vi "sweeper.vi"() -> ()   [LabVIEW 2012]
uses:
  scan_info.ctl
  stimulus.ctl
  injection_point.ctl
  initialization/micron_globals.vi
  <vilib>/Analysis/1siggen.llb/Ramp Pattern by Samples.vi
  <vilib>/Analysis/NI_AALBase.lvlib
panel:
  in  "Axis mode":enum16{"Absolute axis", "Relative axis", "Pose"}(ring)
  in  "Motion axis":string(combo)
  out "Current point":dbl format="%#_3p"
  in  "1/x scaling":bool
  in  "stop":bool
  out "Sweeping":bool
  in  "Linear type":u16(ring) items=["Linear", "Logarithmic"]
  in  "Sweep info":T1 {"End" format="%#_3p"; "Start" format="%#_3p"}
  in  "Start sweep":bool
  in  "Manual":bool
  in  "Stimulus":T2={"Type"=enum."Off", "Phase"=0.0, "Amplitude"=[0.0, 0.0, 0.0, 0.0, 0.0, 0.0], "Injection point"=enum."Total pose", "Closed loop"=TRUE, "Offset"=[0.0, 0.0, 0.0, 0.0, 0.0, 0.0], "Tip -> world"=TRUE, "Frequency"=0.0, "Length"=0.0} {"Length" min=0.0 max=100.0 step=100.0 format="%#_4p"; "Frequency" min=0.0 step=100.0 format="%#_4g"; "Offset" format="%#_3p"; "Amplitude" format="%#_3p"; "Phase" min=-180.0 max=360.0 step=100.0 format="%#.2f"}
  in  "Scrollbar":sgl(c297)
  # "Sweeper"
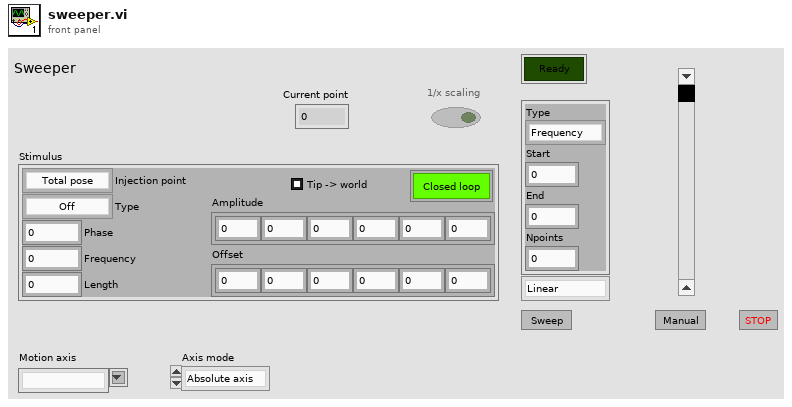
[diagram p1: front panel]
types:
  T1 = typedef "scan_info.ctl" = cluster{"Type":enum16{"Frequency", "Offset", "Motion"}, "Start":sgl, "End":sgl, "Npoints":i32}
  T2 = typedef "stimulus.ctl" = cluster{"Type":enum16{"Off", "Step", "Sine", "Triangle", "Arbitrary"}, "Phase":dbl, "Amplitude":sgl[], "Injection point":T3, "Closed loop":bool, "Offset":sgl[], "Tip -> world":bool, "Frequency":dbl, "Length":dbl}
  T3 = typedef "injection_point.ctl" = enum16{"Total pose", "V limiter", "Goal ", "Link position", "KF link position", "Inverse kin", "Link goal", "Link error", "Controller", "Output", "Drive", "Light"}
  T4 = enum8{"Enabled", "Disabled", "Disabled and Grayed Out"}
  T5 = typedef "ui_override_opts.ctl" = cluster{"Triggering":bool, "Parameters":bool, "Stimulus":bool, "Calibration":bool, "Modes":bool}
  T6 = typedef "Micron params.ctl" = cluster{"Stimulus":T2, "Goal Filter A":T7, "Mode controls":T8, "Manipulator type":enum16{"Current piezo", "Voltage piezo"}, "Manipulator calibration":T9, "Network":T11, "Goal Filter B":T7, "Cancellation":T12, "Transition time":sgl, "Estimation":T14}
  T7 = typedef "goal_loop_parms.ctl" = cluster{"Speedup max":sgl, "Speedup thresh":sgl, "Speedup nonlin":sgl, "Filters":cluster{"Lower Fc":sgl, "Lower Q":sgl, "Scale factor":sgl, "Upper Fc":sgl, "Upper Q":sgl, "V limit":sgl, "V limit range":sgl}[]}
  T8 = typedef "mode_conrols.ctl" = cluster{"Hold":bool, "Cancellation":bool, "Goal filter":bool, "Trigger":bool}
  T9 = typedef "manipulator_cal.ctl" = cluster{"Tool offsets":sgl[][], "Tip light calibration":T10, "Handle light calibration":T10, "Base pivots":sgl[][], "Output pivots":sgl[][], "Length center":sgl, "Workspace height":sgl[], "Workspace diameter":sgl[], "Linearization":sgl[][], "Stack travel":sgl, "Saturation pos":sgl, "Inverse filters":cluster{"filter structure":enum32{"IIR 2nd Order", "IIR 4th Order"}, "Reverse Coefficients":dbl[], "Forward Coefficients":dbl[]}[]}
  T10 = typedef "probe_calibration.ctl" = sgl[][]
  T11 = typedef "network_params.ctl" = cluster{"Remote Host":string, "Send Status":bool, "Send Port":u16, "Recv Commands":bool, "Recv Port":u16}
  T12 = typedef "sq_control_params.ctl" = cluster{"KP":T13, "KI":sgl, "KD":T13, "Max vel":sgl, "Max acc":sgl, "Int error limit":sgl, "RCM gain":sgl, "Bypass":bool, "Degraded gain":sgl}
  T13 = typedef "decoupled_gain.ctl" = cluster{"XY":sgl, "Rxy":sgl, "Z":sgl, "Rz":sgl}
  T14 = typedef "estimation_controls.ctl" = cluster{"Link":cluster{"Measure noise":dbl[], "Process noise":dbl[], "Alt process noise":dbl[], "Alt turnoff cycles":i32, "Innovation limit":dbl[], "Residue threshold":dbl, "Enable":bool}, "Handle":cluster{"Measure noise":dbl[], "Process noise":dbl[], "State limits":dbl[], "Innovation limit":dbl[], "Prediction Lookahead":sgl, "Enable":bool}}
  T15 = typedef "motion_status.ctl" = cluster{"Axis names":string[], "Axis positions":dbl[], "Pose":dbl[], "Timestamp":u32, "Ready":bool, "Stopped":bool}
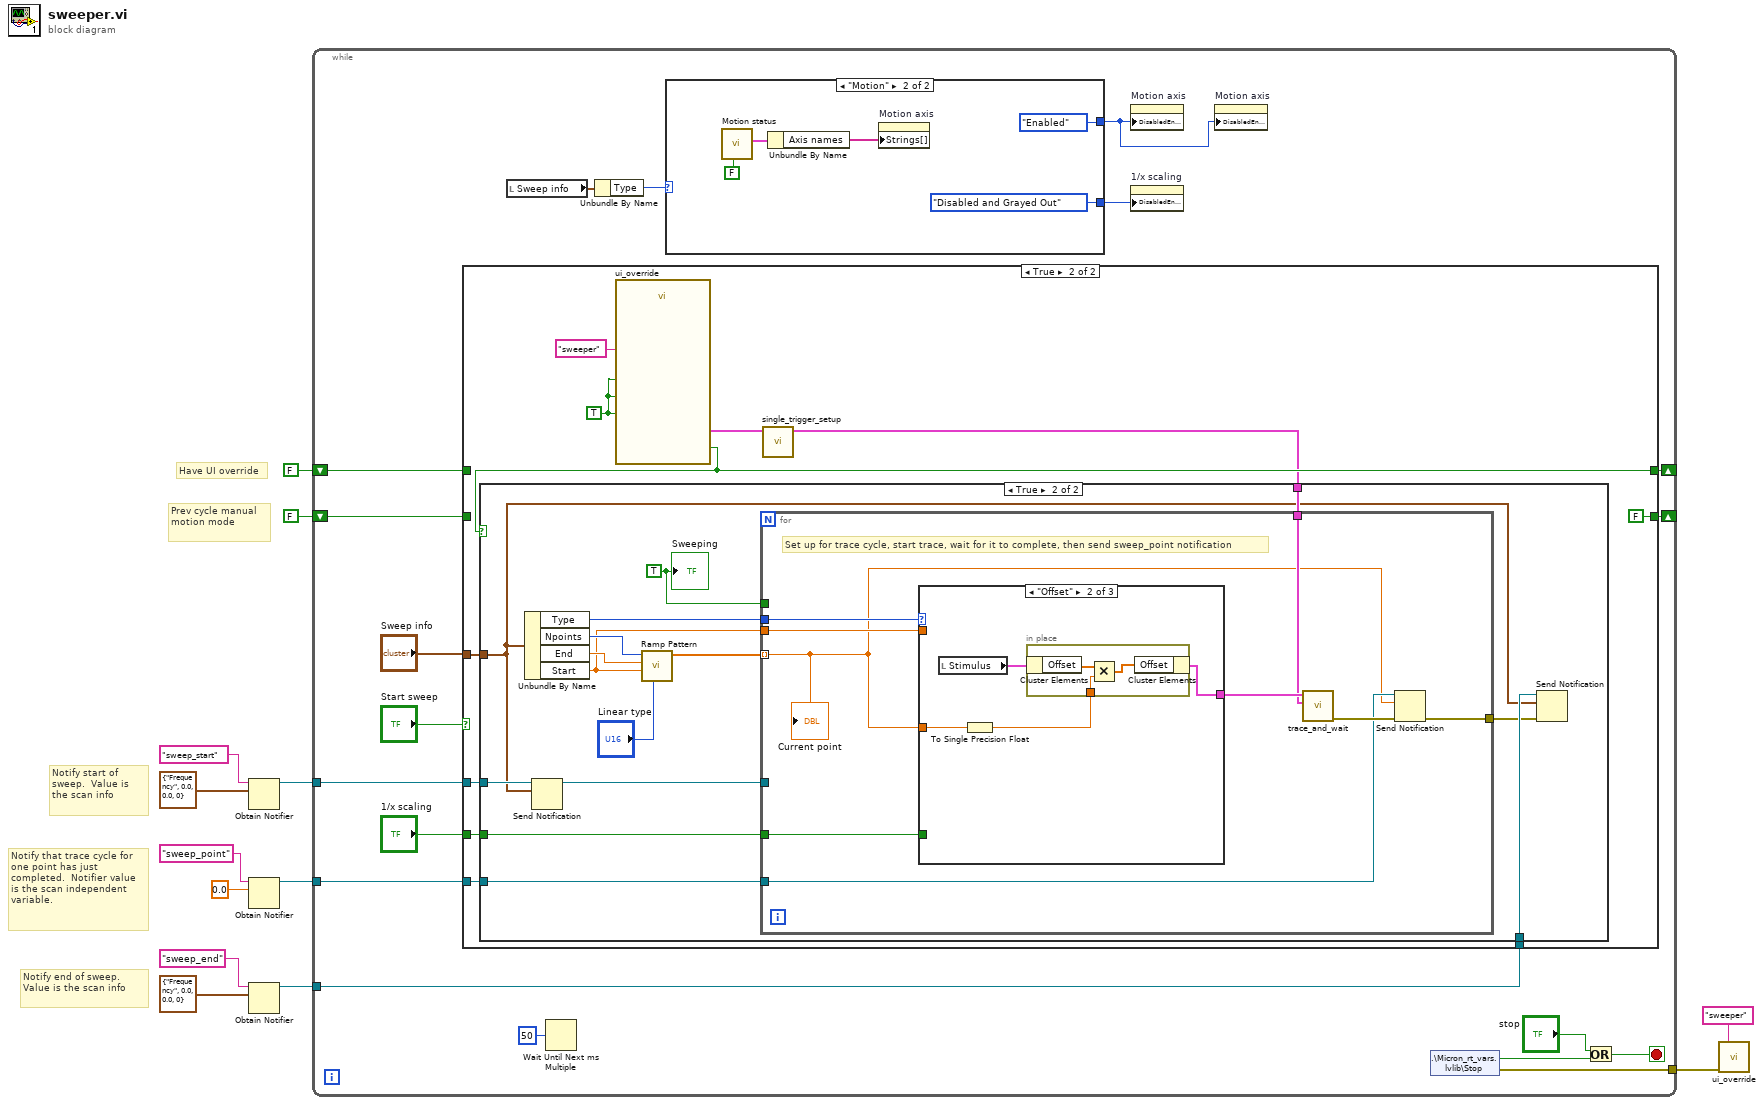
[diagram p0: block diagram]
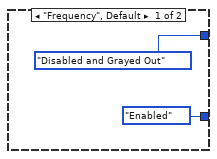
[diagram p2: hidden frame]
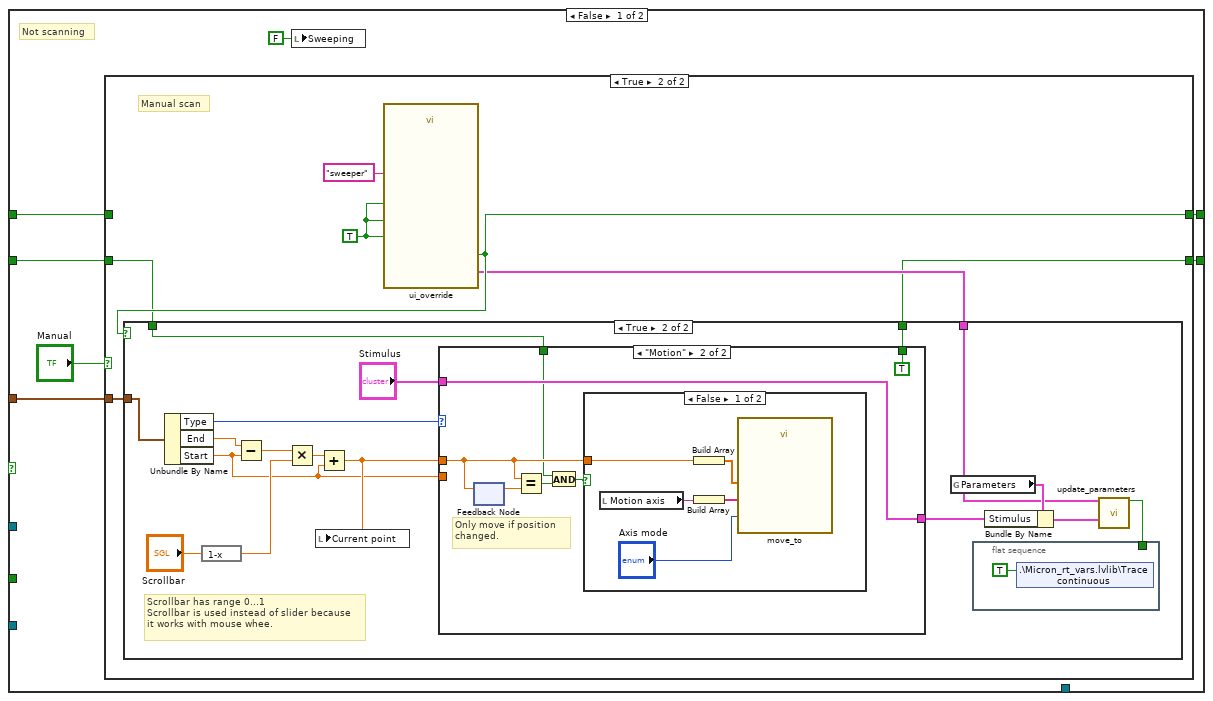
[diagram p3: hidden frame]
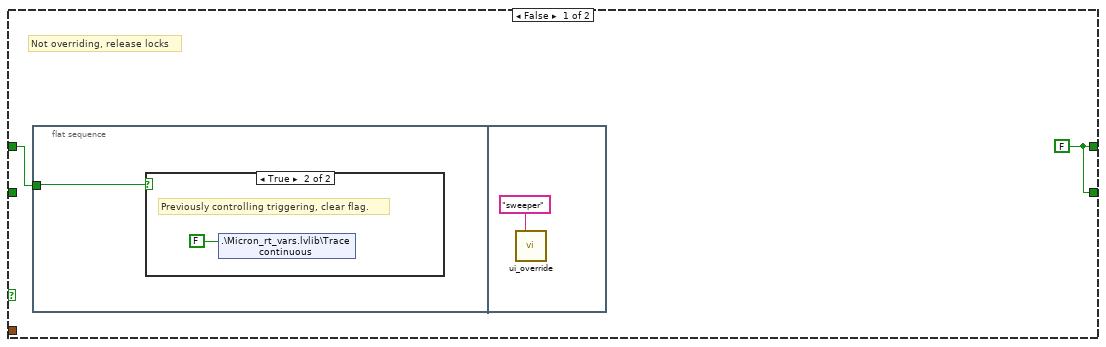
[diagram p4: hidden frame]
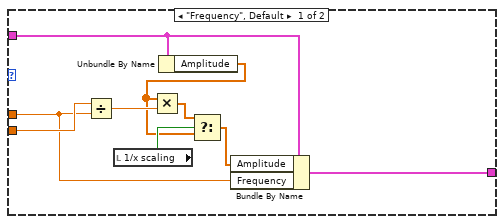
[diagram p7: hidden frame]
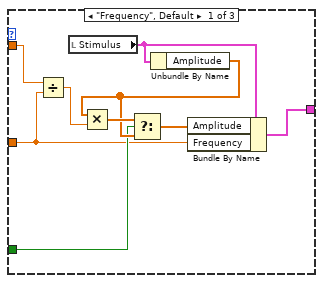
[diagram p10: hidden frame]
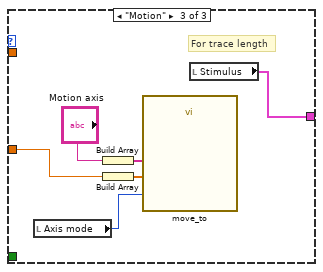
[diagram p11: hidden frame]
diagram:
  # "Prev cycle manual motion mode"
  # "Have UI override"
  # "Notify end of sweep.  Value is the scan info"
  # "Notify that trace cycle for one point has just completed.  Notifier value is the scan independent variable."
  # "Notify start of sweep.  Value is the scan info"
  n1 = Obtain Notifier(name (unnamed)="sweep_start", notification data type=T1 {"Type"=enum."Frequency", "Start"=0.0, "End"=0.0, "Npoints"=0} ("Scan Info")) -> (notifier out=w11:refnum<notifier>)  [unwired: 2 in, 2 out]
  n2 = Obtain Notifier(name (unnamed)="sweep_point", notification data type=0.0) -> (notifier out=w7:refnum<notifier>)  [unwired: 2 in, 2 out]
  n3 = Obtain Notifier(name (unnamed)="sweep_end", notification data type=T1 {"Type"=enum."Frequency", "Start"=0.0, "End"=0.0, "Npoints"=0} ("Scan Info")) -> (notifier out=w4:refnum<notifier>)  [unwired: 2 in, 2 out]
  n4 = while {
    tunnel: w11 -> [w30]
    shift-right: [w24] -> _
    shift-left: FALSE ("Triggering") -> [w23]
    tunnel: w7 -> [w19]
    tunnel: w4 -> [w18]
    tunnel: [w16] -> w2
    shift-right: [w14] -> _
    shift-left: FALSE ("Triggering") -> [w15]
    stop <- w29 stop-if-true
    n5 = case shown="True" "Start sweep" {
      tunnel: "Sweep info" -> [w42 w107]
      tunnel: w30 -> [_ w108]
      tunnel: "1/x scaling" -> [_ w106]
      tunnel: [w44 w103] -> w24
      tunnel: w23 -> [w43 _]
      tunnel: w19 -> [_ w102]
      tunnel: w18 -> [_ w101]
      tunnel: w15 -> [w41 _]
      tunnel: [w40 FALSE ("Triggering")] -> w14
      frame False {
        # "Not scanning"
        n6 = case shown="True" "Manual" {
          tunnel: [w47 w56] -> w44
          tunnel: w43 -> [w48 _]
          tunnel: w42 -> [_ w54]
          tunnel: w41 -> [_ w53]
          tunnel: [w47 w52] -> w40
          frame False {
            w47 = FALSE ("Got all")
            # "Not overriding, release locks"
            n7 = flat-sequence {
              tunnel: w48 -> [w49]
              frame #0 {
                n8 = case shown="True" w49 {
                  frame False {
                  }
                  frame True {
                    # "Previously controlling triggering, clear flag."
                    n9 = shared-variable ".\\Micron_rt_vars.lvlib\\Trace continuous"(FALSE ("UI external stimulus")) -> ()  [unwired: 1 in, 1 out]
                  }
                }
              }
              frame #1 {
                n10 = call "ui_override.vi"("VI name"="sweeper") -> ()  [unwired: 12 in, 3 out]
              }
            }
          }
          frame True {
            w57 = TRUE ("Triggering")
            # "Manual scan"
            n11 = call "ui_override.vi"("Triggering"=w57, "VI name"="sweeper", "Stimulus"=w57, "All or nothing"=w57) -> ("Override"=w55:T5, "Got all"=w56:bool)  [unwired: 9 in, 1 out]
            n12 = case shown="True" w56 {
              tunnel: w55 -> [_ w70]
              tunnel: w54 -> [_ w65]
              tunnel: w53 -> [_ w60]
              tunnel: [_ w59] -> w52
              frame False {
              }
              frame True {
                # "Scrollbar has range 0...1\nScrollbar is used instead of slider because\nit works with mouse whee."
                n13 = Unbundle By Name(w65) -> ("Type"=w64:enum16{"Frequency", "Offset", "Motion"}, "End"=w62:sgl, "Start"=w61:sgl)
                n14 = expression code="1-x"("Scrollbar") -> (w66:sgl)
                n15 = Subtract(x=w62, y=w61) -> (x-y=w69:sgl)
                n16 = Multiply(x=w69, y=w66) -> (x*y=w68:sgl)
                n17 = Add(x=w68, y=w61) -> (x+y=w63:sgl)
                n18 = local write "Current point"(w63) -> ()
                n19 = case shown="\"Motion\"" w64 {
                  tunnel: [w84 w91] -> w73
                  tunnel: "Stimulus" -> [w82 w91]
                  tunnel: w63 -> [w76 w90]
                  tunnel: w61 -> [w77 _]
                  tunnel: w60 -> [_ w87]
                  tunnel: [_ TRUE ("Triggering")] -> w59
                  frame "Frequency", Default {
                    n20 = Divide(x=w77, y=w76) -> (x/y=w80:sgl)
                    n21 = local read "1/x scaling"() -> (w83:bool)
                    n22 = Unbundle By Name(w82) -> ("Amplitude"=w78:sgl[])
                    n23 = Multiply(x=w78, y=w80) -> (x*y=w79:sgl[])
                    n24 = Select(t=w79, s=w83, f=w78) -> (s? t:f=w81:sgl[])
                    n25 = Bundle By Name(cluster=w82, "Amplitude"=w81, "Frequency"=w76) -> (w84:T2)
                  }
                  frame "Motion" {
                    # "Only move if position\nchanged."
                    n26 = feedback-in #1(w90) -> ()
                    n27 = feedback #1() -> (w89:sgl)  [unwired: 1 in]
                    n28 = Equal?(x=w90, y=w89) -> (x = y?=w88:bool)
                    n29 = And(x=w87, y=w88) -> (x .and. y?=w85:bool)
                    n30 = case shown="False" w85 {
                      tunnel: w90 -> [w93 _]
                      frame False {
                        n31 = local read "Motion axis"() -> (w94:string)
                        n32 = Build Array(w93) -> (w96:sgl[])
                        n33 = Build Array(w94) -> (w95:string[])
                        n34 = call "move_to.vi"("Axis names"=w95, "Axis positions"=w96, "Mode"="Axis mode") -> ()  [unwired: 8 in, 1 out]
                      }
                      frame True {
                      }
                    }
                  }
                }
                n35 = global read "micron_globals.vi" "Parameters"() -> (w75:T6)
                n36 = flat-sequence {
                  tunnel: w71 -> [_]
                  frame #0 {
                    n37 = shared-variable ".\\Micron_rt_vars.lvlib\\Trace continuous"(TRUE ("Start trace")) -> ()  [unwired: 1 in, 1 out]
                  }
                }
                n38 = Bundle By Name(cluster=w75, "Stimulus"=w73) -> (w74:T6)
                n39 = call "update_parameters.vi"("Modify"=w70, "Parameters"=w74) -> ("Changed"=w71:bool)  [unwired: 12 in, 1 out]
              }
            }
          }
        }
        n40 = local write "Sweeping"(FALSE ("Scanning")) -> ()
      }
      frame True {
        w104 = TRUE ("Triggering")
        n41 = call "ui_override.vi"("Triggering"=w104, "VI name"="sweeper", "Stimulus"=w104, "All or nothing"=w104) -> ("Override"=w100:T5, "Got all"=w103:bool)  [unwired: 9 in, 1 out]
        n42 = call "single_trigger_setup.vi"("Override in"=w100) -> ("Override out"=w99:T5)  [unwired: 10 in]
        n43 = case shown="True" w103 {
          tunnel: w108 -> [_ w122]
          tunnel: w107 -> [_ w110]
          tunnel: w106 -> [_ w117]
          tunnel: w99 -> [_ w114]
          tunnel: w102 -> [_ w112]
          tunnel: w101 -> [_ w111]
          frame False {
          }
          frame True {
            w115 = TRUE ("Scanning")
            n44 = Unbundle By Name(w110) -> ("Type"=w113:enum16{"Frequency", "Offset", "Motion"}, "Npoints"=w123:i32, "End"=w118:sgl, "Start"=w116:sgl)
            n45 = Send Notification(notification=w110, notifier=w122) -> (notifier out=w120:refnum<notifier>)  [unwired: 1 in, 1 out]
            n46 = call-poly <vilib>:"Ramp Pattern.vi"("type"="Linear type", "start"=w116, "end"=w118, "samples"=w123) -> ("Ramp Pattern"=w121:dbl[])  [unwired: 6 in, 1 out]
            n47 = for {
              tunnel: w121 -> [w124] mode=indexing
              tunnel: w120 -> [_]
              tunnel: w116 -> [w131]
              tunnel: w117 -> [w132]
              tunnel: w115 -> [_]
              tunnel: w114 -> [w127]
              tunnel: w113 -> [w130]
              tunnel: w112 -> [w126]
              tunnel: [w125] -> w109
              # "Set up for trace cycle, start trace, wait for it to complete, then send sweep_point notification"
              n48 = case shown="\"Offset\"" w130 {
                tunnel: w132 -> [w138 _ _]
                tunnel: w131 -> [w136 _ _]
                tunnel: w124 -> [w135 w144 w153]
                tunnel: [w133 w142 w150] -> w128
                frame "Frequency", Default {
                  n49 = Divide(x=w136, y=w135) -> (x/y=w134:dbl)
                  n50 = local read "Stimulus"() -> (w141:T2)
                  n51 = Unbundle By Name(w141) -> ("Amplitude"=w139:sgl[])
                  n52 = Multiply(x=w139, y=w134) -> (x*y=w140:dbl[])
                  n53 = Select(t=w140, s=w138, f=w139) -> (s? t:f=w137:dbl[])
                  n54 = Bundle By Name(cluster=w141, "Amplitude"=w137, "Frequency"=w135) -> (w133:T2)
                }
                frame "Offset" {
                  n55 = local read "Stimulus"() -> (w145:T2)
                  n56 = To Single Precision Float(number=w144) -> (single precision float=w143:sgl)
                  n57 = in-place {
                    in-place-border: w143 -> [w147]
                    n58 = in-place-cluster #2(w145) -> ("Offset"=w148:sgl[])
                    n59 = Multiply(x=w148, y=w147) -> (x*y=w146:sgl[])
                    n60 = in-place-cluster #2("Offset"=w146) -> (w142:T2)
                  }
                }
                frame "Motion" {
                  # "For trace length"
                  n61 = local read "Axis mode"() -> (w149:enum16{"Absolute axis", "Relative axis", "Pose"})
                  n62 = Build Array("Motion axis") -> (w151:string[])
                  n63 = Build Array(w153) -> (w152:dbl[])
                  n64 = call "move_to.vi"("Axis names"=w151, "Axis positions"=w152, "Mode"=w149) -> ()  [unwired: 8 in, 1 out]
                  n65 = local read "Stimulus"() -> (w150:T2)
                }
              }
              n66 = call "trace_and_wait.vi"("Override"=w127, "Stimulus"=w128) -> ("error out"=w129:errorcluster)  [unwired: 9 in]
              n67 = Send Notification(notification=w124, notifier=w126, error in (no error)=w129) -> (error out=w125:errorcluster)  [unwired: 1 out]
              "Current point" <- w124
            }
            n68 = Send Notification(notification=w110, notifier=w111, error in (no error)=w109) -> ()  [unwired: 2 out]
            "Sweeping" <- w115
          }
        }
      }
    }
    n69 = local read "Sweep info"() -> (w22:T1)
    n70 = Wait Until Next ms Multiple(millisecond multiple=u32 50) -> ()  [unwired: 1 out]
    n71 = Unbundle By Name(w22) -> ("Type"=w21:enum16{"Frequency", "Offset", "Motion"})
    n72 = case shown="\"Motion\"" w21 {
      tunnel: [T4."Enabled" ("Disabled") T4."Disabled and Grayed Out" ("Disabled")] -> w20
      tunnel: [T4."Disabled and Grayed Out" ("Disabled") T4."Enabled" ("Disabled")] -> w17
      frame "Frequency", Default {
      }
      frame "Motion" {
        n73 = call "Motion status.vi"("Wait for updated value (F)"=FALSE ("Wait for updated value (T)")) -> ("Motion status"=w37:T15)  [unwired: 5 in, 5 out]
        n74 = Unbundle By Name(w37) -> ("Axis names"=w35:string[])
        n75 = property on="Motion axis" class="CmbBox"("Strings[]"=w35) -> ()  [unwired: 2 in, 2 out]
      }
    }
    n76 = property on="Motion axis" class="CmbBox"("DisabledEnum"=w17) -> ()  [unwired: 2 in, 2 out]
    n77 = property on="1/x scaling" class="Bool (strict)"("DisabledEnum"=w20) -> ()  [unwired: 2 in, 2 out]
    n78 = property on="Motion axis" class="CmbBox"("DisabledEnum"=w17) -> ()  [unwired: 2 in, 2 out]
    n79 = shared-variable ".\\Micron_rt_vars.lvlib\\Stop"() -> (w27:bool, error out=w16:errorcluster)  [unwired: 1 in]
    n80 = Or(x="stop", y=w27) -> (x .or. y?=w29:bool)
  }
  n81 = call "ui_override.vi"("VI name"="sweeper", "error in"=w2) -> ()  [unwired: 11 in, 3 out]
